vi "Displayspeed.vi"() -> (1 "Increment":dbl, 2 "DisplaySpeed":dbl, 3 "Waitin(ms)":dbl)   [LabVIEW 2016]
uses:
  Globaltracker.vi
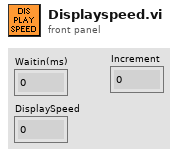
[diagram p1: front panel]
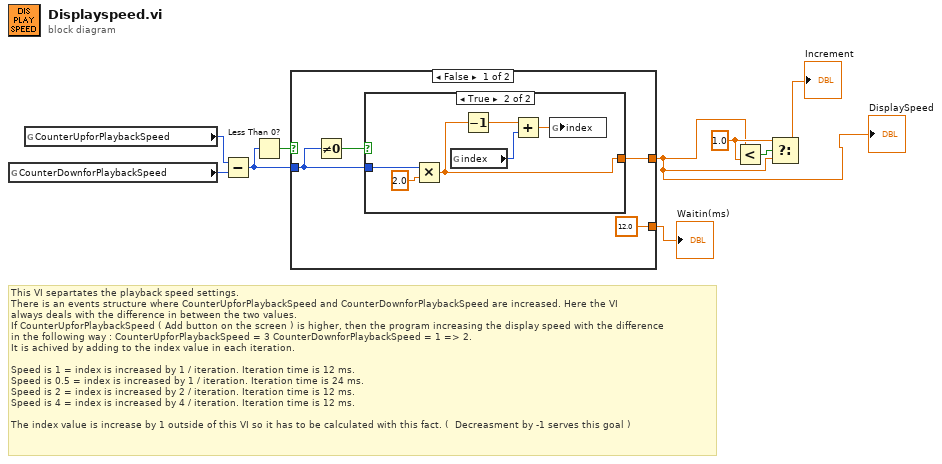
[diagram p0: block diagram]
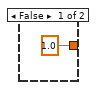
[diagram p2: hidden frame]
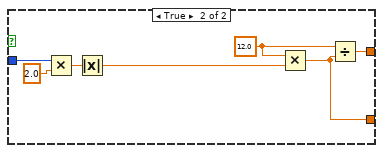
[diagram p3: hidden frame]
diagram:
  w3 = 1.0 ("x")
  # "This VI separtates the playback speed settings. \nThere is an events structure where CounterUpforPlaybackSpeed and CounterDownforPlaybackSpeed are increased. Here the VI\nalways deals with the difference in between the two values. \nIf CounterUpforPlaybackSpeed ( Add button on the screen ) is higher, then the program increasing the display speed with the difference \nin the following way : CounterUpforPlaybackSpeed = 3 CounterDownforPlaybackSpeed = 1 => 2. \nIt is achived by adding to the index value in each iteration. \n\nSpeed is 1 = index is increased by 1 / iteration. Iteration time is 12 ms.\nSpeed is 0.5 = index is increased by 1 / iteration. Iteration time is 24 ms.\nSpeed is 2 = index is increased by 2 / iteration. Iteration time is 12 ms. \nSpeed is 4 = index is increased by 4 / iteration. Iteration time is 12 ms. \n\nThe index value is increase by 1 outside of this VI so it has to be calculated with this fact. (  Decreasment by -1 serves this goal )"
  n1 = global read "Globaltracker.vi" "CounterDownforPlaybackSpeed"() -> (w9:i16)
  n2 = global read "Globaltracker.vi" "CounterUpforPlaybackSpeed"() -> (w8:i16)
  n3 = Subtract(x=w8, y=w9) -> (x-y=w5:i16)
  n4 = Less Than 0?(x=w5) -> (x < 0?=w6:bool)
  n5 = case shown="False" w6 {
    tunnel: [12.0 w25] -> w7
    tunnel: w5 -> [w11 w24]
    tunnel: [w10 w21] -> w2
    frame False {
      n6 = Not Equal To 0?(x=w11) -> (x != 0?=w12:bool)
      n7 = case shown="True" w12 {
        tunnel: w11 -> [_ w19]
        tunnel: [1.0 ("_Speed_") w15] -> w10
        frame False {
        }
        frame True {
          n8 = Multiply(x=w19, y=2.0) -> (x*y=w15:dbl)
          n9 = global read "Globaltracker.vi" "index"() -> (w17:i16)
          n10 = Decrement(x=w15) -> (x-1=w18:dbl)
          n11 = Add(x=w18, y=w17) -> (x+y=w16:dbl)
          n12 = global write "Globaltracker.vi" "index"(w16) -> ()
        }
      }
    }
    frame True {
      w26 = 12.0 ("x")
      n13 = Multiply(x=w24, y=2.0) -> (x*y=w22:dbl)
      n14 = Absolute Value(x=w22) -> (abs(x)=w27:dbl)
      n15 = Multiply(x=w26, y=w27) -> (x*y=w25:dbl)
      n16 = Divide(x=w26, y=w25) -> (x/y=w21:dbl)
    }
  }
  "Waitin(ms)" <- w7
  "DisplaySpeed" <- w2
  n17 = Less?(x=w2, y=w3) -> (x < y?=w4:bool)
  n18 = Select(t=w3, s=w4, f=w2) -> (s? t:f=→"Increment":dbl)
